vi "Get HW Interface Outputs.vi"(8 "error in (no error)":errorcluster, 11 "Hardware Interface in":refnum<class "Hardware Interface.lvclass">) -> (0 "error out":errorcluster, 1 "Digital Outputs":T1, 2 "Analog Outputs":T2, 3 "Hardware Interface out":refnum<class "Hardware Interface.lvclass">)   [LabVIEW 2013, in "Hardware Interface.lvclass"]
uses:
  Hardware Interface.lvclass
  DblArrayWithName.ctl
  BoolArrayWithName.ctl
  Hardware Interface.lvclass/Hardware Interface.ctl
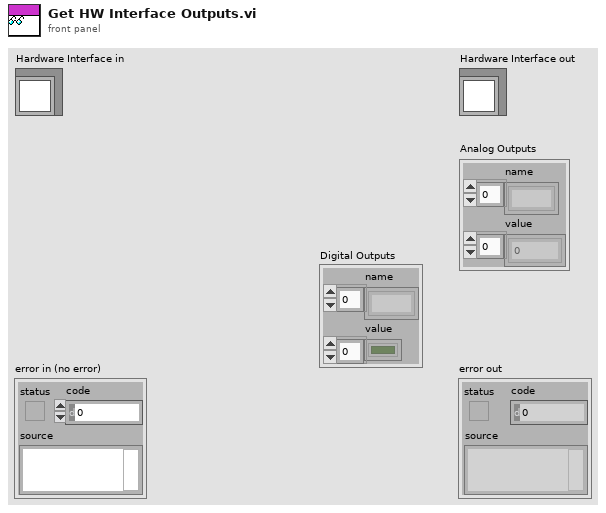
[diagram p1: front panel]
types:
  T1 = typedef "BoolArrayWithName.ctl" = cluster{"name":string[], "value":bool[]}
  T2 = typedef "DblArrayWithName.ctl" = cluster{"name":string[], "value":dbl[]}
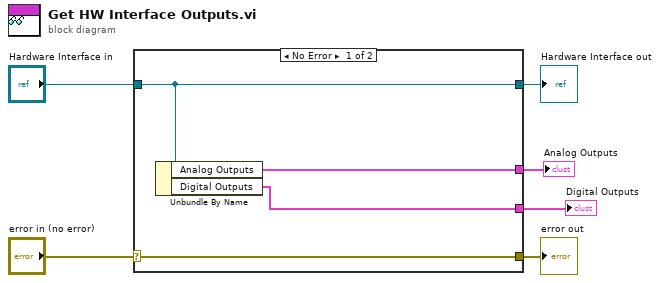
[diagram p0: block diagram]
diagram:
  n1 = case shown="No Error" "error in (no error)" {
    selector: "error in (no error)" -> [w10 w11]
    tunnel: [w10 w11] -> w5
    tunnel: [w9 w12] -> w3
    tunnel: "Hardware Interface in" -> [w9 w12]
    tunnel: [w8 _] -> w2
    tunnel: [w7 _] -> w1
    frame No Error {
      n2 = Unbundle By Name(w9) -> ("Analog Outputs"=w8:T2, "Digital Outputs"=w7:T1)
    }
    frame Error {
    }
  }
  "error out" <- w5
  "Hardware Interface out" <- w3
  "Analog Outputs" <- w2
  "Digital Outputs" <- w1
